vi "Async.Processes.Report.vi"(8 "Error":errorcluster, 10 "Stop Async on Error?":bool, 11 "Process in":refnum<class "Process.lvclass">) -> (2 "Stop":bool, 3 "Process out":refnum<class "Process.lvclass">)   [LabVIEW 2015, in "VS Inline Async API.lvlib" / "Process.lvclass"]
uses:
  Process.lvclass
  Process.lvclass/Process.ctl
  VS Inline Async API.lvlib
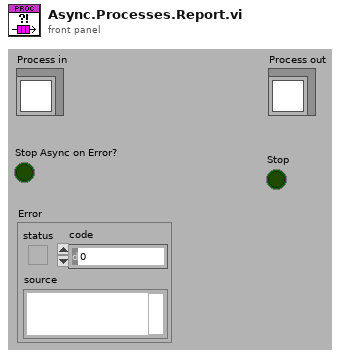
[diagram p1: front panel]
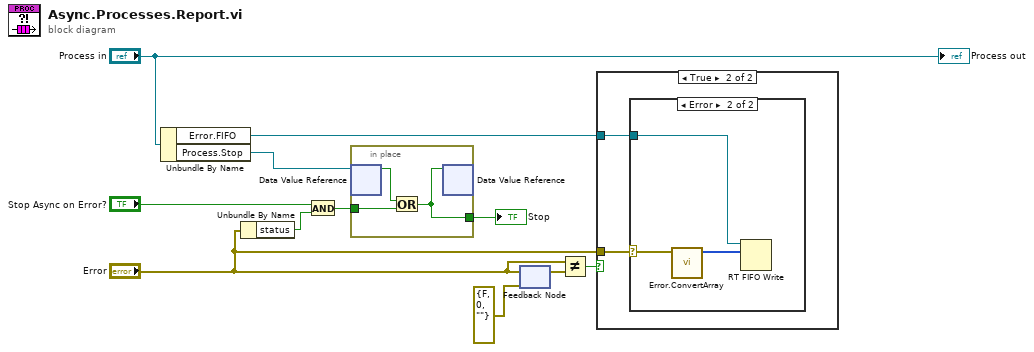
[diagram p0: block diagram]
diagram:
  n1 = Unbundle By Name("Process in") -> ("Error.FIFO"=w8:refnum<k33>, "Process.Stop"=w2:refnum<data-value>)
  n2 = Unbundle By Name("Error") -> ("status"=w6:bool)
  n3 = And(x="Stop Async on Error?", y=w6) -> (x .and. y?=w5:bool)
  n4 = in-place {
    in-place-border: [w12] -> w4
    in-place-border: w5 -> [w13]
    n5 = in-place-dvr #1(w2) -> (w14:bool)  [unwired: 1 out]
    n6 = Or(x=w14, y=w13) -> (x .or. y?=w12:bool)
    n7 = in-place-dvr #1(w12) -> ()  [unwired: 2 out]
  }
  "Stop" <- w4
  n8 = feedback #2(errorcluster {"status"=FALSE, "code"=0, "source"=""} ("Error")) -> (w10:errorcluster)
  n9 = feedback-in #2("Error") -> ()
  n10 = Not Equal?(x="Error", y=w10) -> (x != y?=w11:bool)
  n11 = case shown="True" w11 {
    tunnel: w8 -> [_ w16]
    tunnel: "Error" -> [_ w15]
    frame False {
    }
    frame True {
      n12 = case shown="Error" w15 {
        selector: w15 -> [_ w18]
        tunnel: w16 -> [_ w19]
        frame No Error {
        }
        frame Error {
          n13 = call "Error.ConvertArray.vi"("error in"=w18) -> ("Msg"=w17:u8[])  [unwired: 10 in]
          n14 = RT FIFO Write(0:w19, 1:w17) -> ()  [unwired: 3 in, 4 out]
        }
      }
    }
  }
  "Process out" <- "Process in"
